vi "Dashboard Main.vi"() -> ()   [LabVIEW 2011]
uses:
  <vilib>/Rock Robotics/WPI/Camera/WPI_CameraImageSize.ctl
  <vilib>/Rock Robotics/WPI/DriverStation/WPI_DriverStationDigitalData.ctl
  <vilib>/Rock Robotics/WPI/Camera/WPI_CameraWhite Balance Values.ctl
  <vilib>/vision/NI_Vision_Development_Module.lvlib
panel:
  out "fps":dbl
  in  "x":u32=500
  in  "Camera Settings":T2={"FPS"=10, "Compression"=30, "Image Size"=enum."320x240"}
  out "Processed Image":T3(plugin-control)
  out "Original Image":T3(plugin-control)
  in  "Annotate":bool=TRUE
  in  "Processing":enum32{"Color", "Intensity", "Intensity Open"}(tab)
  in  "Luminance":i32=255
  in  "Saturation":i32=255
  in  "Hue":i32(knob)=65 scale=0.0..255.0
  in  "Margins":cluster{"Hue":i32, "Sat":i32, "Lum":i32}={"Hue"=9, "Sat"=40, "Lum"=19} {"Sat" scale=0.0..40.0; "Lum" scale=0.0..40.0; "Hue" scale=0.0..40.0}
  in  "Range":cluster{"Lower value":sgl, "Upper value":sgl}={"Lower value"=150.0, "Upper value"=255.0} {"Lower value" scale=0.0..255.0; "Upper value" scale=0.0..255.0}
  in  "Range 2":cluster{"Lower value":sgl, "Upper value":sgl}={"Lower value"=150.0, "Upper value"=255.0} {"Lower value" scale=0.0..255.0; "Upper value" scale=0.0..255.0}
  out "Target Info":T4(array[cluster])
  in  "Particle Count Limit":i32=10
  in  "Area Size Limit":i32=444
  in  "Score Limits":T5={"Rect Coverage"=76.0, "Aspect Ratio"=70.0, "X Edge Strength"=40.0, "Y Edge Strength"=60.0}
  in  "Camera Type":enum16{"206", "1011"}(ring)
  in  "Viewer":enum32{"Camera Image", "Kinect Skeleton"}(tab)
  in  "Video Enable":bool=TRUE
  out "Camera Image":T3(plugin-control)
  out "Buttons 1":cluster{"1":bool, "2":bool, "3":bool}
  out "Kinect 1":cluster{"X":dbl, "Y":dbl, "Z":dbl} {"X" scale=1.0..-1.0; "Y" scale=1.0..-1.0; "Z" scale=1.0..-1.0}
  out "Buttons 2":cluster{"1":bool, "2":bool, "3":bool}
  out "Kinect 2":cluster{"X":dbl, "Y":dbl, "Z":dbl} {"X" scale=1.0..-1.0; "Y" scale=1.0..-1.0; "Z" scale=1.0..-1.0}
  out "Version":string
  out "Skeleton Picture":picture
  out "Players":i8
  out "Dashboard Datatype Warning":string="Warning: The Dashboard Datatype used by the robot project and this dashboard do not match.\nSee diagram for more details."
  out "Robot IP Address":string
  out "Image Error Message":string="Timeout in Camera Communications"
  # "Communications"
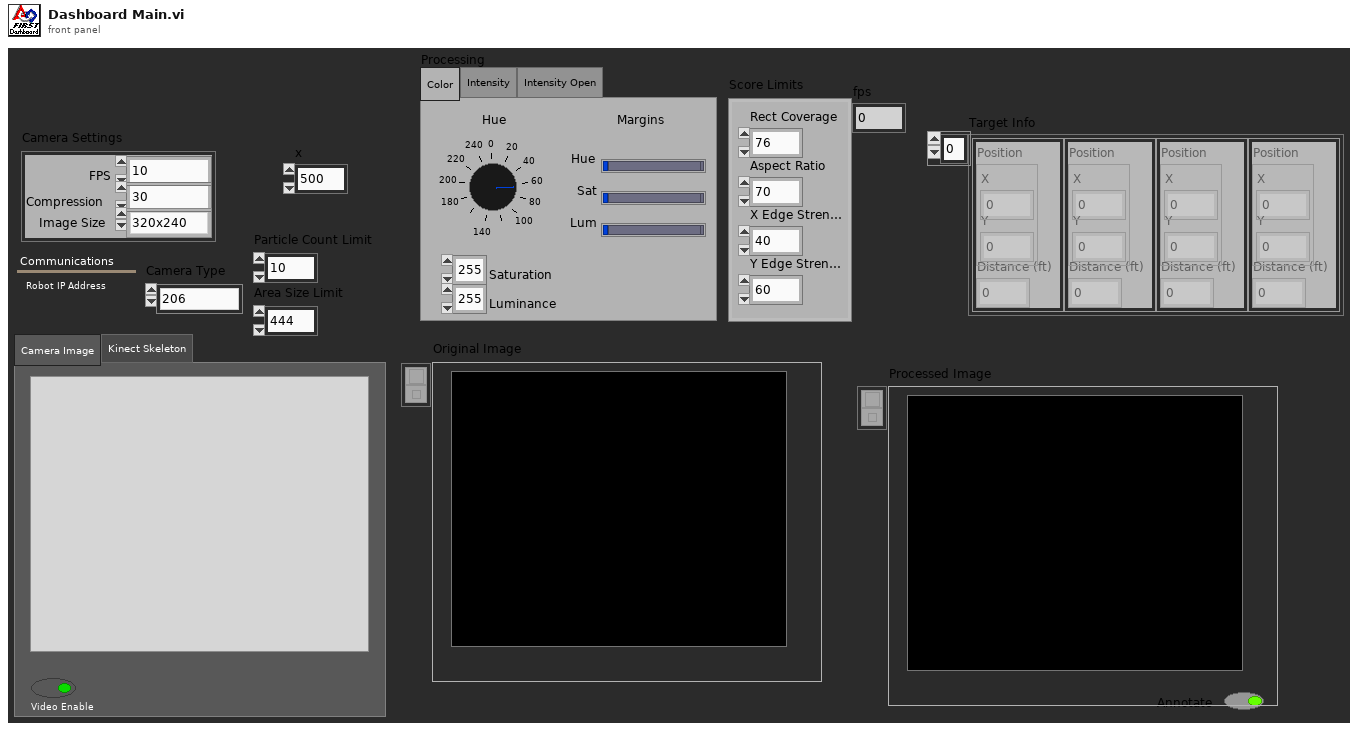
[diagram p1: front panel]
types:
  T1 = typedef "WPI_CameraImageSize.ctl" = enum16{"640x480", "320x240", "160x120"}
  T2 = cluster{"FPS":i32, "Compression":i32, "Image Size":T1}
  T3 = typedef "IMAQ Image.ctl" = refnum<image>
  T4 = cluster{"Position":cluster{"X":dbl, "Y":dbl}, "Distance (ft)":dbl}[]
  T5 = cluster{"Rect Coverage":dbl, "Aspect Ratio":dbl, "X Edge Strength":dbl, "Y Edge Strength":dbl}
  T6 = typedef "WPI_CameraWhite Balance Values.ctl" = enum16{"Auto", "Fixed indoor", "Fixed outdoor 1", "Fixed outdoor 2", "Fixed fluorescent 1", "Fixed fluorescent 2", "Hold current"}
  T7 = typedef "Image Type" = u32
  T8 = typedef "WPI_DriverStationDigitalData.ctl" = cluster{"Relay Fwd":u8, "Relay Rev":u8, "GPIO":u16, "GPIO_OE":u16, "PWM":cluster{"PWM[0]":u8, "PWM[1]":u8, "PWM[2]":u8, "PWM[3]":u8, "PWM[4]":u8, "PWM[5]":u8, "PWM[6]":u8, "PWM[7]":u8, "PWM[8]":u8, "PWM[9]":u8}}
  T9 = cluster{cluster{"AnalogModule[0]":cluster{"Channel[0]":sgl, "Channel[1]":sgl, "Channel[2]":sgl, "Channel[3]":sgl, "Channel[4]":sgl, "Channel[5]":sgl, "Channel[6]":sgl, "Channel[7]":sgl}, "AnalogModule[1]":cluster{"Channel[0]":sgl, "Channel[1]":sgl, "Channel[2]":sgl, "Channel[3]":sgl, "Channel[4]":sgl, "Channel[5]":sgl, "Channel[6]":sgl, "Channel[7]":sgl}}, cluster{"DigitalModule[0]":T8, "DigitalModule[1]":T8}, "Solenoid":u8}
  T10 = typedef "WPI_CameraDevRef.ctl" = cluster{"Camera Address":string, "CameraStatus":errorcluster, "Acquire Image Notifier":refnum<notifier>}
  T11 = cluster{"Left":dbl, "Top":dbl, "Right":dbl, "Bottom":dbl}
  T12 = enum32{"AutoM", "Close", "Dilate", "Erode", "Gradient", "Gradient out", "Gradient in", "Hit miss", "Open", "PClose", "POpen", "Thick", "Thin"}
  T13 = cluster{cluster{"Left":dbl, "Top":dbl, "Right":dbl, "Bottom":dbl}, dbl[]}[]
  T14 = cluster{"Target Center (-1 to 1)":cluster{"X":dbl, "Y":dbl}, "Distance (ft)":dbl}
  T15 = cluster{"Target Center (-1 to 1)":cluster{"X":dbl, "Y":dbl}, "Distance (ft)":dbl}[]
  T16 = cluster{"Competition mode":bool, "Robot Link":bool, "Autonomous":bool, "Enabled":bool, "E-Stop":bool}
  T17 = cluster{"AnalogModule[0]":cluster{"Channel[0]":sgl, "Channel[1]":sgl, "Channel[2]":sgl, "Channel[3]":sgl, "Channel[4]":sgl, "Channel[5]":sgl, "Channel[6]":sgl, "Channel[7]":sgl}, "AnalogModule[1]":cluster{"Channel[0]":sgl, "Channel[1]":sgl, "Channel[2]":sgl, "Channel[3]":sgl, "Channel[4]":sgl, "Channel[5]":sgl, "Channel[6]":sgl, "Channel[7]":sgl}}
  T18 = cluster{"DigitalModule[0]":T8, "DigitalModule[1]":T8}
  T19 = cluster{"Channel[0]":sgl, "Channel[1]":sgl, "Channel[2]":sgl, "Channel[3]":sgl, "Channel[4]":sgl, "Channel[5]":sgl, "Channel[6]":sgl, "Channel[7]":sgl}[]
  T20 = cluster{"Channel[0]":sgl, "Channel[1]":sgl, "Channel[2]":sgl, "Channel[3]":sgl, "Channel[4]":sgl, "Channel[5]":sgl, "Channel[6]":sgl, "Channel[7]":sgl}
  T21 = typedef "LVRectTypeDef.ctl" = cluster{"left":i16, "top":i16, "right":i16, "bottom":i16}
  T22 = typedef "LVBoundsTypeDef.ctl" = cluster{"Width":u32, "Height":u32}
  T23 = typedef "SkeletonTrackState.ctl" = enum32{"NotTracked", "PositionOnly", "Tracked"}
  T24 = cluster{"TrackingState":u8[], "Position":cluster{"x":sgl, "y":sgl, "z":sgl}, cluster{"x":sgl, "y":sgl, "z":sgl, sgl}[], "TrackState":T23}
  T25 = cluster{cluster{"ScaledToPercentRange":dbl, "ScaledToPercentRange":dbl, "ScaledToPercentRange":dbl}, cluster{bool, bool, bool}}[]
  T26 = cluster{cluster{"ScaledToPercentRange":dbl, "ScaledToPercentRange":dbl, "ScaledToPercentRange":dbl}, cluster{bool, bool, bool}}
  T27 = cluster{"ScaledToPercentRange":dbl, "ScaledToPercentRange":dbl, "ScaledToPercentRange":dbl}
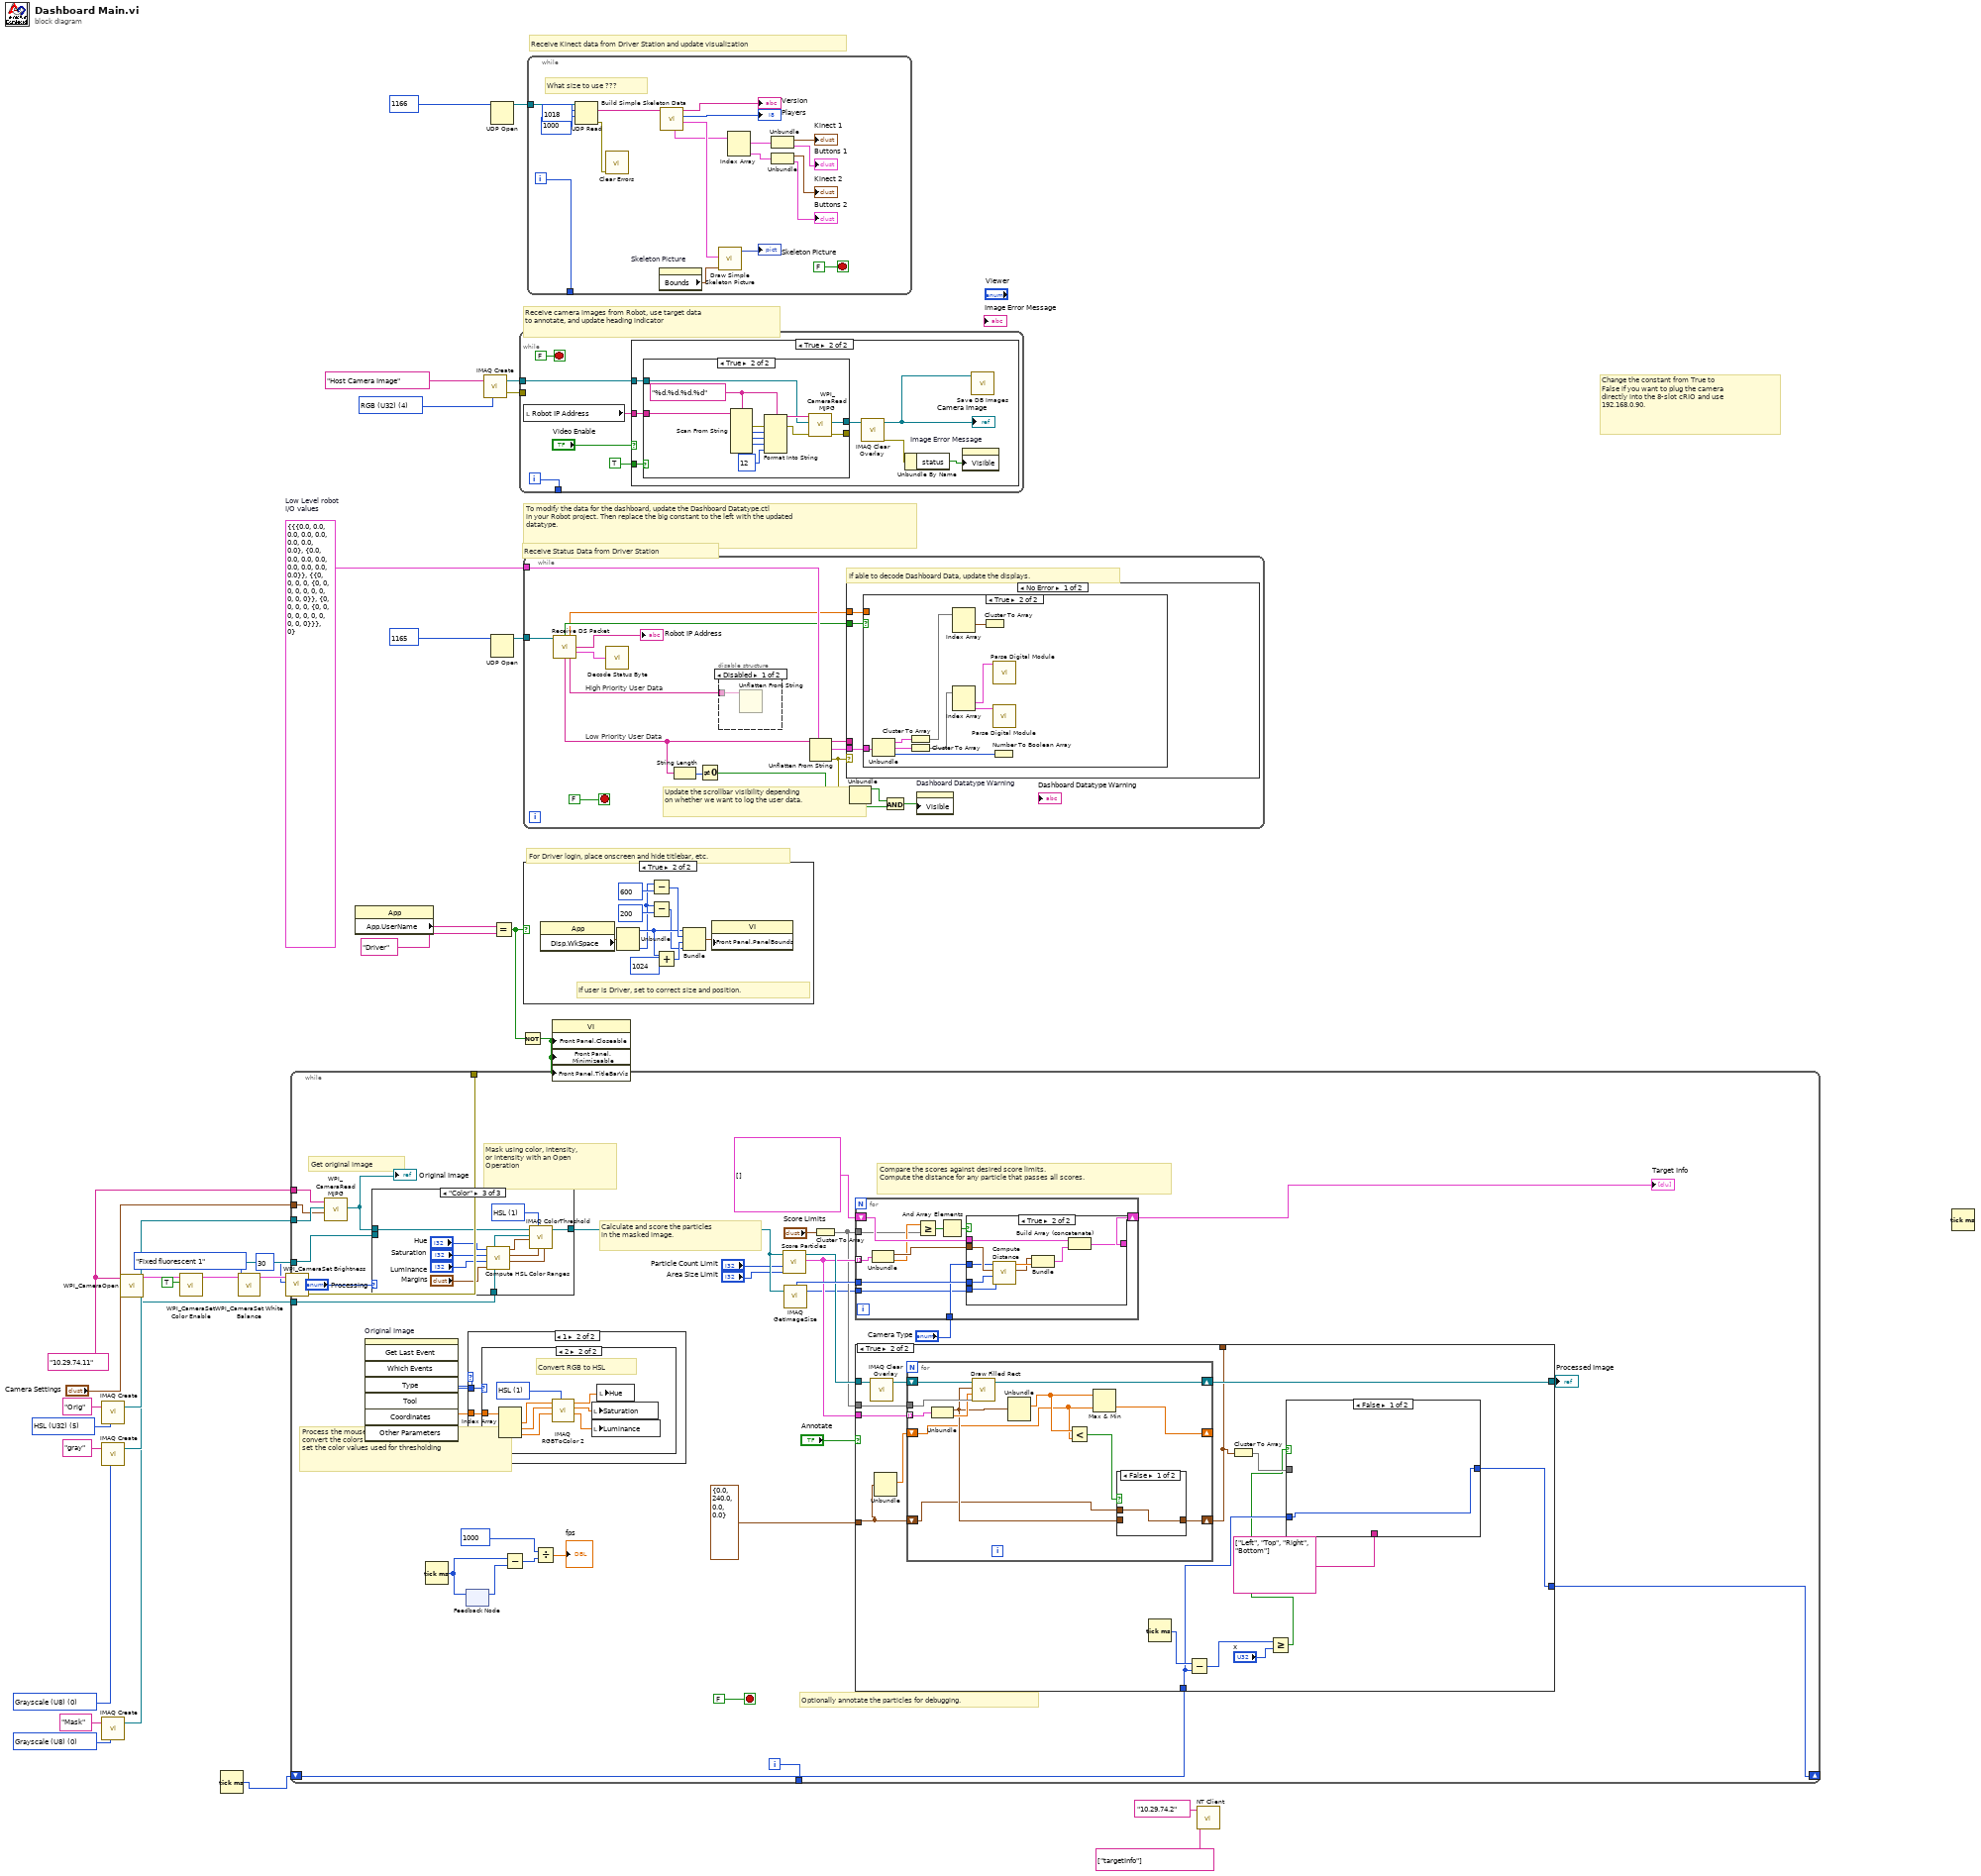
[diagram p0: block diagram]
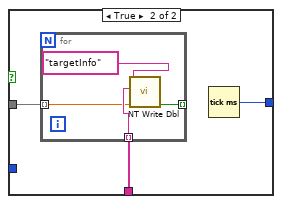
[diagram p3: hidden frame]
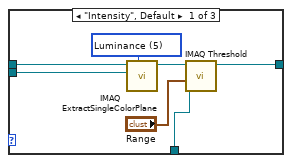
[diagram p5: hidden frame]
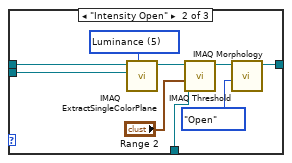
[diagram p6: hidden frame]
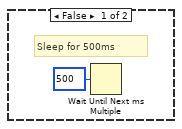
[diagram p14: hidden frame]
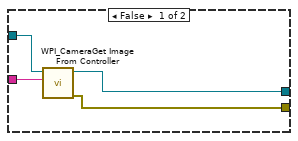
[diagram p15: hidden frame]
diagram:
  w12 = "10.29.74.11" ("Camera IP Address")
  w14 = T7 0 items=["Grayscale (U8)", "Grayscale (I16)", "Grayscale (SGL)", "Complex (CSG)", "RGB (U32)", "HSL (U32)", "RGB (U64)", "Grayscale (U16)"] ("Image Type")
  w18 = T7 5 items=["Grayscale (U8)", "Grayscale (I16)", "Grayscale (SGL)", "Complex (CSG)", "RGB (U32)", "HSL (U32)", "RGB (U64)", "Grayscale (U16)"] ("Image Type")
  w21 = T7 0 items=["Grayscale (U8)", "Grayscale (I16)", "Grayscale (SGL)", "Complex (CSG)", "RGB (U32)", "HSL (U32)", "RGB (U64)", "Grayscale (U16)"] ("Image Type")
  w24 = T9 {{"AnalogModule[0]"={"Channel[0]"=0.0, "Channel[1]"=0.0, "Channel[2]"=0.0, "Channel[3]"=0.0, "Channel[4]"=0.0, "Channel[5]"=0.0, "Channel[6]"=0.0, "Channel[7]"=0.0}, "AnalogModule[1]"={"Channel[0]"=0.0, "Channel[1]"=0.0, "Channel[2]"=0.0, "Channel[3]"=0.0, "Channel[4]"=0.0, "Channel[5]"=0.0, "Channel[6]"=0.0, "Channel[7]"=0.0}}, {"DigitalModule[0]"={"Relay Fwd"=0, "Relay Rev"=0, "GPIO"=0, "GPIO_OE"=0, "PWM"={"PWM[0]"=0, "PWM[1]"=0, "PWM[2]"=0, "PWM[3]"=0, "PWM[4]"=0, "PWM[5]"=0, "PWM[6]"=0, "PWM[7]"=0, "PWM[8]"=0, "PWM[9]"=0}}, "DigitalModule[1]"={"Relay Fwd"=0, "Relay Rev"=0, "GPIO"=0, "GPIO_OE"=0, "PWM"={"PWM[0]"=0, "PWM[1]"=0, "PWM[2]"=0, "PWM[3]"=0, "PWM[4]"=0, "PWM[5]"=0, "PWM[6]"=0, "PWM[7]"=0, "PWM[8]"=0, "PWM[9]"=0}}}, "Solenoid"=0}  # Low Level robot I/O values
  w32 = T7 4 items=["Grayscale (U8)", "Grayscale (I16)", "Grayscale (SGL)", "Complex (CSG)", "RGB (U32)", "HSL (U32)", "RGB (U64)"] ("Image Type")
  # "Change the constant from True to\nFalse if you want to plug the camera\ndirectly into the 8-slot cRIO and use\n192.168.0.90."
  # "Receive Kinect data from Driver Station and update visualization"
  # "For Driver login, place onscreen and hide titlebar, etc."
  # "To modify the data for the dashboard, update the Dashboard Datatype.ctl\nin your Robot project. Then replace the big constant to the left with the updated\ndatatype."
  # "Receive Status Data from Driver Station"
  # "Receive camera images from Robot, use target data\nto annotate, and update heading indicator"
  n1 = call "IMAQ Create"("Image Name"="Orig", "Image Type"=w18) -> ("New Image"=w17:T3)  [unwired: 2 in, 2 out]
  n2 = call "IMAQ Create"("Image Name"="gray", "Image Type"=w21) -> ("New Image"=w16:T3)  [unwired: 2 in, 2 out]
  n3 = call "IMAQ Create"("Image Name"="Mask", "Image Type"=w14) -> ("New Image"=w13:T3)  [unwired: 2 in, 2 out]
  n4 = call <vilib>:"WPI_CameraOpen.vi"("Camera Address"=w12) -> ("CameraDevRef"=w11:T10)  [unwired: 9 in, 1 out]
  n5 = call <vilib>:"WPI_CameraSet Color Enable.vi"("Color Enabled"=TRUE, "CameraDevRef"=w11) -> ("CameraDevRef Out"=w9:T10)  [unwired: 8 in, 1 out]
  n6 = Tick Count (ms)() -> (millisecond timer value=w1:u32)
  n7 = call <vilib>:"WPI_CameraSet White Balance.vi"("White Balance"=WPI_CameraWhite_Balance_Values."Fixed fluorescent 1", "CameraDevRef"=w9) -> ("CameraDevRef Out"=w7:T10)  [unwired: 8 in, 1 out]
  n8 = call <vilib>:"WPI_CameraSet Brightness.vi"("Brightness"=30, "CameraDevRef"=w7) -> ("error out"=w5:errorcluster)  [unwired: 8 in, 1 out]
  n9 = while {
    tunnel: w17 -> [w59]
    tunnel: w16 -> [w68]
    tunnel: w13 -> [w67]
    tunnel: w12 -> [w57]
    tunnel: w5 -> [_]
    tunnel: "Camera Settings" -> [w44]
    shift-right: [w41] -> _
    shift-left: w1 -> [w42]
    tunnel: [w40] -> _
    i -> [w40]
    stop <- FALSE stop-if-true
    # "Optionally annotate the particles for debugging."
    # "Compare the scores against desired score limits.\nCompute the distance for any particle that passes all scores."
    # "Process the mouse click in original image,\nconvert the colors of that pixel to HSL, and\nset the color values used for thresholding"
    # "Calculate and score the particles\nin the masked image."
    # "Mask using color, intensity,\nor intensity with an Open\nOperation"
    # "Get original image"
    n10 = call <vilib>:"WPI_CameraRead MJPG.vi"("Camera Settings"=w44, "Image"=w59, "address"=w57) -> ("Image Out"=w58:T3)  [unwired: 7 in, 1 out]
    "Original Image" <- w58
    n11 = invoke on="Original Image" class="ImageControl" method="Get Last Event"() -> ("Type"=w61:i32, "Tool"=w62:i32, "Other Parameters"=w63:sgl[])  [unwired: 8 in, 5 out]
    n12 = case shown="\"Color\"" "Processing" {
      tunnel: w58 -> [w116 w125 w136]
      tunnel: w68 -> [w115 w124 _]
      tunnel: w67 -> [w113 w122 w135]
      tunnel: [w111 w118 w134] -> w49
      frame "Intensity", Default {
        w110 = 5 items=["Red", "Green", "Blue", "Hue", "Saturation", "Luminance", "Value", "Intensity"] ("Color Plane")
        n13 = call "IMAQ ExtractSingleColorPlane"("Color Plane"=w110, "Image Dst"=w115, "Image Src"=w116) -> ("Image Dst Out"=w114:T3)  [unwired: 1 in, 7 out]
        n14 = call "IMAQ Threshold"("Range"="Range", "Image Dst"=w113, "Image Src"=w114) -> ("Image Dst Out"=w111:T3)  [unwired: 3 in, 5 out]
      }
      frame "Intensity Open" {
        w117 = 5 items=["Red", "Green", "Blue", "Hue", "Saturation", "Luminance", "Value", "Intensity"] ("Color Plane")
        n15 = call "IMAQ ExtractSingleColorPlane"("Color Plane"=w117, "Image Dst"=w124, "Image Src"=w125) -> ("Image Dst Out"=w123:T3)  [unwired: 1 in, 7 out]
        n16 = call "IMAQ Threshold"("Range"="Range 2", "Image Dst"=w122, "Image Src"=w123) -> ("Image Dst Out"=w119:T3)  [unwired: 3 in, 5 out]
        n17 = call "IMAQ Morphology"("Operation"=T12."Open", "Image Src"=w119) -> ("Image Dst Out"=w118:T3)  [unwired: 8 in, 1 out]
      }
      frame "Color" {
        w133 = u16 1 items=["RGB", "HSL", "HSV", "HSI"] ("Color Mode")
        n18 = call "Compute HSL Color Ranges.vi"("Margins"="Margins", "Luminance"="Luminance", "Saturation"="Saturation", "Hue"="Hue") -> ("Lum Range"=w130:cluster{i32, i32}, "Sat Range"=w131:cluster{i32, i32}, "Hue Range"=w132:cluster{i32, i32})  [unwired: 5 in]
        n19 = call "IMAQ ColorThreshold"("Blue or Luma or Val or Inten Range"=w130, "Green or Sat Range"=w131, "Color Mode"=w133, "Red or Hue Range"=w132, "Image Dst"=w135, "Image Src"=w136) -> ("Image Dst Out"=w134:T3)  [unwired: 4 in, 1 out]
      }
    }
    n20 = Tick Count (ms)() -> (millisecond timer value=w38:u32)
    n21 = feedback-in #1(w38) -> ()
    n22 = feedback #1() -> (w39:u32)  [unwired: 1 in]
    n23 = case shown="1" w61 {
      tunnel: w62 -> [_ w159]
      tunnel: w63 -> [_ w158]
      frame 0, Default {
      }
      frame 1 {
        n24 = case shown="2" w159 {
          tunnel: w158 -> [_ w167]
          frame Default {
          }
          frame 2 {
            w166 = u16 1 items=["RGB", "HSL", "HSV", "HSI", "CIE L*a*b*", "CIE XYZ"] ("Color Mode")
            # "Convert RGB to HSL"
            n25 = Index Array(array=w167) -> (element #1=w165:sgl, element #2=w163:sgl, element #3=w161:sgl)  [unwired: 3 in]
            n26 = call "IMAQ RGBToColor 2"("Color Mode"=w166, "Blue value"=w161, "Green value"=w163, "Red value"=w165) -> ("Blue or Luma or Val or Inten or Z or b*value"=w160:dbl, "Green or Sat or Y or a* value"=w162:dbl, "Red or Hue or X or L* value"=w164:dbl)  [unwired: 4 in, 1 out]
            n27 = local write "Saturation"(w162) -> ()
            n28 = local write "Luminance"(w160) -> ()
            n29 = local write "Hue"(w164) -> ()
          }
        }
      }
    }
    n30 = Subtract(x=w38, y=w39) -> (x-y=w37:u32)
    n31 = Divide(x=1000, y=w37) -> (x/y=→"fps":dbl)
    n32 = call "Score Particles.vi"("Area Size Limit"="Area Size Limit", "Particle Count Limit"="Particle Count Limit", "Image Refnum in"=w49) -> ("Scored Particle Info"=w52:T13, "Image Refnum out"=w56:T3)  [unwired: 7 in]
    n33 = call "IMAQ GetImageSize"("Image"=w49) -> ("Y Resolution"=w45:i32, "X Resolution"=w60:i32)  [unwired: 3 in, 1 out]
    n34 = Cluster To Array(cluster="Score Limits") -> (array=w50:dbl[])
    n35 = for {
      shift-right: [w146] -> w64
      shift-left: T4 [] -> [w147]
      tunnel: w60 -> [w145]
      tunnel: w52 -> [w143] mode=indexing
      tunnel: w50 -> [w138]
      tunnel: "Camera Type" -> [w142]
      tunnel: w45 -> [w137]
      n36 = Unbundle(w143) -> (w144:T11, w139:dbl[])
      n37 = Greater Or Equal?(x=w139, y=w138) -> (x >= y?=w141:bool[])
      n38 = And Array Elements(Boolean array=w141) -> (logical AND=w140:bool)
      n39 = case shown="True" w140 {
        tunnel: w147 -> [w148 w157]
        tunnel: [w148 w156] -> w146
        tunnel: w144 -> [_ w152]
        tunnel: w145 -> [_ w154]
        tunnel: w142 -> [_ w151]
        tunnel: w137 -> [_ w149]
        frame False {
        }
        frame True {
          n40 = call "Compute Distance.vi"("Y Image Resolution"=w149, "X Image Resolution"=w154, "Bounding Box"=w152, "Camera Type"=w151) -> ("Target Center (-1 to 1)"=w150:cluster{"X":dbl, "Y":dbl}, "Distance (ft)"=w153:dbl)  [unwired: 6 in]
          n41 = Bundle("Target Center (-1 to 1)"=w150, "Distance (ft)"=w153) -> (w155:T14)  [unwired: 1 in]
          n42 = Build Array (concatenate)(w157, w155) -> (w156:T15)
        }
      }
    }
    "Target Info" <- w64
    n43 = case shown="True" "Annotate" {
      tunnel: w56 -> [w71 w87]
      tunnel: [w71 w86] -> w53
      tunnel: w52 -> [_ w84]
      tunnel: w50 -> [_ w83]
      tunnel: [w70 w80] -> _
      tunnel: T11 {"Left"=0.0, "Top"=240.0, "Right"=0.0, "Bottom"=0.0} -> [w70 w82]
      tunnel: w42 -> [w69 w73]
      tunnel: [w69 w74] -> w41
      frame False {
      }
      frame True {
        n44 = call "IMAQ Clear Overlay"("Image"=w87) -> ("Image Out"=w85:T3)  [unwired: 2 in, 8 out]
        n45 = Unbundle(w82) -> ("Top"=w81:dbl)  [unwired: 3 out]
        n46 = for {
          shift-right: [w106] -> w86
          shift-left: w85 -> [w107]
          tunnel: w84 -> [w105] mode=indexing
          tunnel: w83 -> [w104]
          shift-right: [w99] -> _
          shift-left: w81 -> [w97]
          shift-right: [w101] -> w80
          shift-left: w82 -> [w100]
          n47 = Unbundle(w105) -> (w102:T11, w103:dbl[])
          n48 = call "Draw Filled Rect.vi"("Limits"=w104, "Scores"=w103, "Bounding Box"=w102, "image in"=w107) -> ("image out"=w106:T3)  [unwired: 7 in]
          n49 = Unbundle(w102) -> ("Top"=w98:dbl)  [unwired: 3 out]
          n50 = Less?(x=w98, y=w97) -> (x < y?=w96:bool)
          n51 = Max & Min(x=w98, y=w97) -> (min(x,y)=w99:dbl)  [unwired: 1 out]
          n52 = case shown="False" w96 {
            tunnel: w102 -> [_ w109]
            tunnel: [w108 w109] -> w101
            tunnel: w100 -> [w108 _]
            frame False {
            }
            frame True {
            }
          }
        }
        n53 = Tick Count (ms)() -> (millisecond timer value=w77:u32)
        n54 = Subtract(x=w77, y=w73) -> (x-y=w76:u32)
        n55 = Cluster To Array(cluster=w80) -> (array=w78:dbl[])
        n56 = Greater Or Equal?(x=w76, y="x") -> (x >= y?=w72:bool)
        n57 = case shown="False" w72 {
          tunnel: string[] ["Left", "Top", "Right", "Bottom"] ("Requested Tables") -> [_ w91]
          tunnel: w78 -> [_ w90]
          tunnel: [w88 w89] -> w74
          tunnel: w73 -> [w88 _]
          frame False {
          }
          frame True {
            n58 = for {
              tunnel: w91 -> [w95] mode=indexing
              tunnel: w90 -> [w94] mode=indexing
              tunnel: [w92] -> _ mode=indexing
              n59 = call "NT Write Dbl.vi"("Dbl"=w94, "Field"=w95, "Table"="targetInfo") -> ("Success"=w92:bool)  [unwired: 7 in, 1 out]
            }
            n60 = Tick Count (ms)() -> (millisecond timer value=w89:u32)
          }
        }
      }
    }
    "Processed Image" <- w53
  }
  n61 = property class="App"() -> ("App.UserName"=w27:string)  [unwired: 2 in, 2 out]
  n62 = call "IMAQ Create"("Image Name"="Host Camera Image", "Image Type"=w32) -> ("New Image"=w30:T3, "error out"=w29:errorcluster)  [unwired: 2 in, 1 out]
  n63 = UDP Open(11:u16 1166 ("port")) -> (port=w22:refnum<k16>)  [unwired: 2 in, 4 out]
  n64 = UDP Open(11:u16 1165 ("port")) -> (port=w33:refnum<k16>)  [unwired: 2 in, 4 out]
  n65 = Equal?(x=w27, y="Driver") -> (x = y?=w26:bool)
  n66 = while {
    tunnel: w30 -> [w171]
    tunnel: w29 -> [_]
    tunnel: [w168] -> _
    i -> [w168]
    stop <- FALSE stop-if-true
    n67 = local read "Robot IP Address"() -> (w172:string)
    n68 = case shown="True" "Video Enable" {
      tunnel: w172 -> [_ w181]
      tunnel: w171 -> [_ w180]
      tunnel: TRUE -> [_ w175]
      frame False {
        # "Sleep for 500ms"
        n69 = Wait Until Next ms Multiple(millisecond multiple=u32 500) -> ()  [unwired: 1 out]
      }
      frame True {
        n70 = case shown="True" w175 {
          tunnel: w180 -> [w184 w191]
          tunnel: [w182 w189] -> _
          tunnel: [w183 w190] -> w177
          tunnel: w181 -> [w185 w194]
          frame False {
            n71 = call <vilib>:"WPI_CameraGet Image From Controller.vi"("Controller Address"=w185, "Image"=w184) -> ("error out"=w182:errorcluster, "Image Out"=w183:T3)  [unwired: 2 in, 6 out]
          }
          frame True {
            w186 = "%d.%d.%d.%d" ("format string")
            n72 = Scan From String(format string=w186, input string=w194) -> (error out=w193:errorcluster, output 1=w195:i32, output 2=w196:i32, output 3=w197:i32)  [unwired: 2 in, 7 out]
            n73 = Format Into String(format string=w186, error in=w193, w195, w196, w197, 12 ("IP Suffix:")) -> (resulting string=w192:string, error out=w188:errorcluster)  [unwired: 1 in]
            n74 = call <vilib>:"WPI_CameraRead MJPG.vi"("error in"=w188, "Image"=w191, "address"=w192) -> ("error out"=w189:errorcluster, "Image Out"=w190:T3)  [unwired: 7 in]
          }
        }
        n75 = call "IMAQ Clear Overlay"("Image"=w177) -> ("error out"=w178:errorcluster, "Image Out"=w176:T3)  [unwired: 2 in, 7 out]
        "Camera Image" <- w176
        n76 = Unbundle By Name(w178) -> ("status"=w179:bool)
        n77 = property on="Image Error Message" class="Str"("Visible"=w179) -> ()  [unwired: 2 in, 2 out]
        n78 = call "Save DB Images.vi"("Image"=w176) -> ()  [unwired: 2 in, 1 out]
      }
    }
  }
  n79 = Not(x=w26) -> (.not. x?=w25:bool)
  n80 = while {
    tunnel: w33 -> [w211]
    tunnel: w24 -> [w210]
    stop <- FALSE stop-if-true
    # "High Priority User Data"
    # "Low Priority User Data"
    # "Update the scrollbar visibility depending\non whether we want to log the user data."
    # "If able to decode Dashboard Data, update the displays."
    n81 = call "Receive DS Packet.vi"("Recv Socket"=w211) -> ("New Dashboard Data"=w207:bool, "Battery"=w198:sgl, "Robot IP Address"=→"Robot IP Address":string, "Status"=w212:T16, "Low Priority User Data"=w200:string, "High Priority User Data"=w199:string)  [unwired: 1 in, 8 out]
    n82 = call "Decode Status Byte.vi"("Status Byte"=w212) -> ()  [unwired: 2 out]
    n83 = String Length(string=w200) -> (length=w202:i32)
    n84 = Not Equal To 0?(x=w202) -> (x != 0?=w205:bool)
    n85 = disable-structure shown="Disabled" {
      disable-tunnel: w199 -> [w214 _]
      frame Disabled {
        n86 = Unflatten From String(binary string=w214) -> ()  [unwired: 2 in, 5 out]
      }
      frame Enabled {
      }
    }
    n87 = Unflatten From String(type=w210, binary string=w200) -> (rest of the binary string=w203:string, value=w209:T9, error out=w208:errorcluster)  [unwired: 1 in, 2 out]
    n88 = case shown="No Error" w208 {
      tunnel: w209 -> [w217 _]
      tunnel: w207 -> [w216 _]
      tunnel: w203 -> [_ _]
      tunnel: w198 -> [w215 _]
      frame No Error {
        n89 = case shown="True" w216 {
          tunnel: w217 -> [_ w222]
          tunnel: w215 -> [_ _]
          frame False {
            # "Don't update if the robot hasn't sent new data"
          }
          frame True {
            n90 = Unbundle(w222) -> (w219:T17, w220:T18, "Solenoid"=w221:u8)
            n91 = Cluster To Array(cluster=w219) -> (array=w226:T19)
            n92 = Cluster To Array(cluster=w220) -> (array=w225:T8[])
            n93 = Index Array(array=w226) -> (element #1=w218:T20)  [unwired: 2 in, 1 out]
            n94 = Index Array(array=w225) -> (element #1=w224:T8, element #2=w223:T8)  [unwired: 2 in]
            n95 = Cluster To Array(cluster=w218) -> ()  [unwired: 1 out]
            n96 = call "Parse Digital Module.vi"("DigitalModule"=w223) -> ()  [unwired: 11 out]
            n97 = Number To Boolean Array(number=w221) -> ()  [unwired: 1 out]
            n98 = call "Parse Digital Module.vi"("DigitalModule"=w224) -> ()  [unwired: 11 out]
          }
        }
      }
      frame Error {
        # "Your datatypes don't match. The Dashboard Datatype.ctl in your Robot project\nand the big constant to the left of the loop need to match."
      }
    }
    n99 = Unbundle(w208) -> ("status"=w204:bool)  [unwired: 2 out]
    n100 = And(x=w204, y=w205) -> (x .and. y?=w206:bool)
    n101 = property on="Dashboard Datatype Warning" class="Str"("Visible"=w206) -> ()  [unwired: 2 in, 2 out]
  }
  n102 = case shown="True" w26 {
    frame False {
    }
    frame True {
      # "If user is Driver, set to correct size and position."
      n103 = property class="App"() -> ("Disp.WkSpace"=w236:T21)  [unwired: 2 in, 2 out]
      n104 = Unbundle(w236) -> ("left"=w231:i16, "bottom"=w227:i16)  [unwired: 2 out]
      n105 = Subtract(x=w227, y=600) -> (x-y=w233:i32)
      n106 = Subtract(x=w227, y=200) -> (x-y=w228:i32)
      n107 = Add(x=w231, y=1024) -> (x+y=w232:i32)
      n108 = Bundle("left"=w231, w233, w232, w228) -> (w235:cluster{"left":i16, i32, i32, i32})  [unwired: 1 out]
      n109 = property class="VI"("Front Panel.PanelBounds"=w235) -> ()  [unwired: 2 in, 2 out]
    }
  }
  n110 = while {
    tunnel: w22 -> [w253]
    tunnel: [w237] -> _
    i -> [w237]
    stop <- FALSE stop-if-true
    # "What size to use ???"
    n111 = UDP Read(connection ID=w253, max size (548)=1018 ("bytes to read"), timeout ms (25000)=1000) -> (data out=w247:string, error out=w245:errorcluster)  [unwired: 1 in, 3 out]
    n112 = call <vilib>:"Clear Errors.vi"("error in (no error)"=w245) -> ()  [unwired: 6 in, 1 out]
    n113 = property on="Skeleton Picture" class="Pict"() -> ("Bounds"=w249:T22)  [unwired: 2 in, 2 out]
    n114 = call "Build Simple Skeleton Data.vi"("data out"=w247) -> ("Skeleton Data"=w248:T24, "NumPlayers"=→"Players":i8, "Version String"=→"Version":string, "Simple Joystick Info"=w244:T25)  [unwired: 6 in, 1 out]
    n115 = call "Draw Simple Skeleton Picture.vi"("Bounds"=w249, "Simple Skeleton"=w248) -> ("new picture out"=→"Skeleton Picture":picture)  [unwired: 9 in]
    n116 = Index Array(array=w244) -> (element #1=w243:T26, element #2=w242:T26)  [unwired: 2 in]
    n117 = Unbundle(w243) -> (→"Kinect 1":T27, →"Buttons 1":cluster{bool, bool, bool})
    n118 = Unbundle(w242) -> (→"Kinect 2":T27, →"Buttons 2":cluster{bool, bool, bool})
  }
  n119 = property class="VI"("Front Panel.Closeable"=w25, "Front Panel.Minimizeable"=w25, "Front Panel.TitleBarVis"=w25) -> ()  [unwired: 2 in, 2 out]
  n120 = call "NT Client.vi"("Requested Tables"=string[] ["targetInfo"], "server IP Address"="10.29.74.2") -> ()  [unwired: 10 in]
  n121 = Tick Count (ms)() -> ()  [unwired: 1 out]
